vi "Alarms FGV.vi"(6 "Alarms Info":T1, 7 "Function":enum16{"Read", "Write", "Clear"}(ring)) -> (2 "Alarms Info Out":T1)   [LabVIEW 2020]
uses:
  Alarms Info Cluster.ctl
panel:
  out "error out":errorcluster
  in  "error in":errorcluster
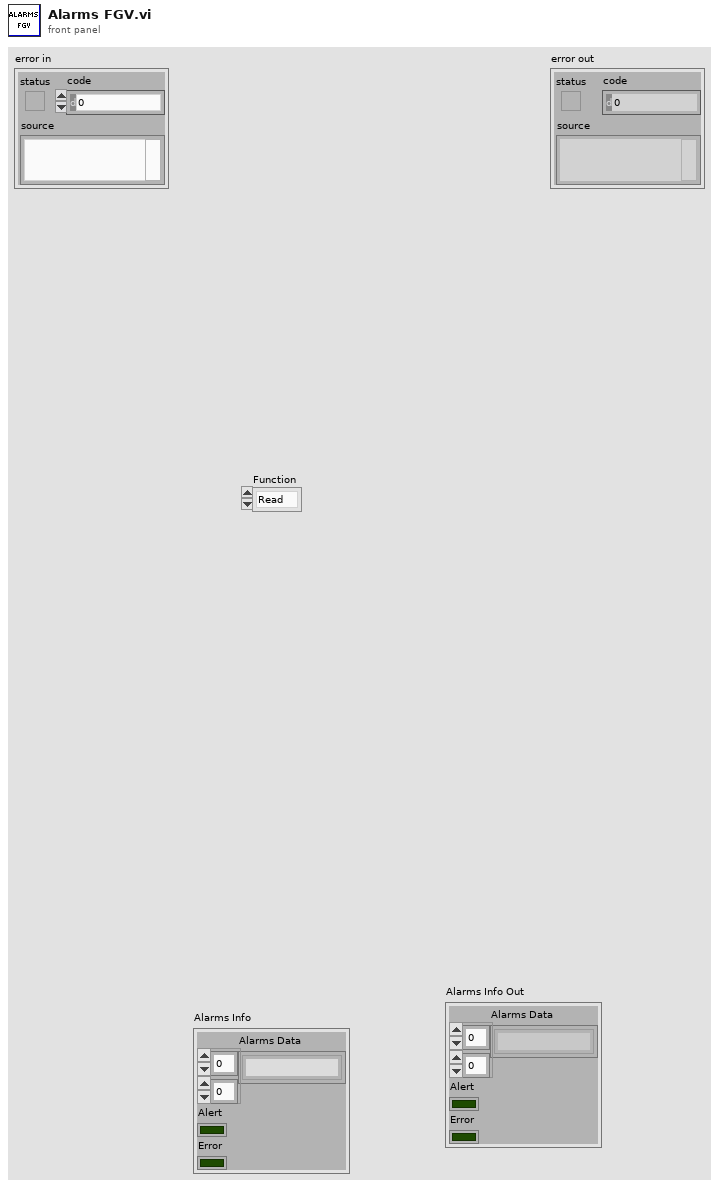
[diagram p1: front panel]
types:
  T1 = typedef "Alarms Info Cluster.ctl" = cluster{"Alarms Data":string[][], "Alert":bool, "Error":bool}
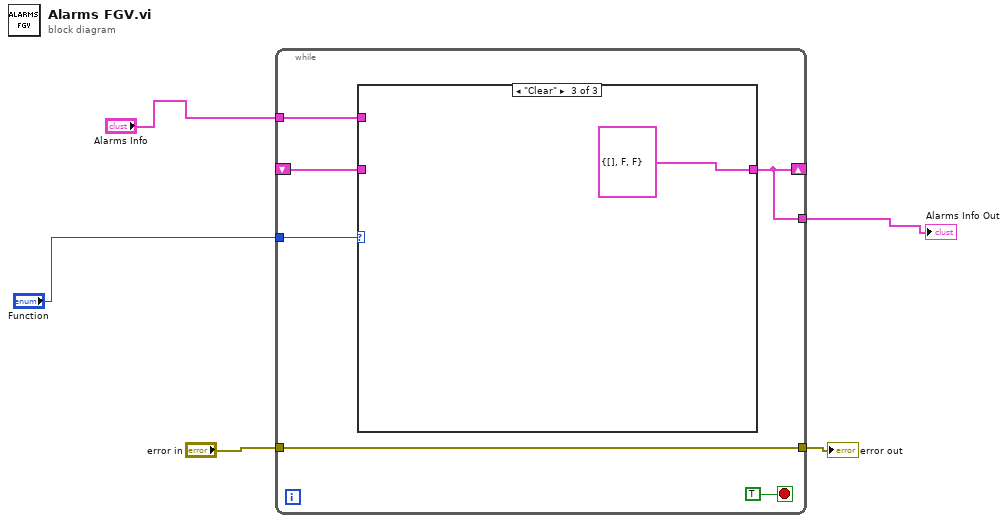
[diagram p0: block diagram]
diagram:
  n1 = while {
    tunnel: "Function" -> [w10]
    shift-right: [w7] -> _
    shift-left: _ -> [w8]
    tunnel: "Alarms Info" -> [w9]
    tunnel: [w7] -> w2
    tunnel: "error in" -> [w6]
    tunnel: [w6] -> w3
    stop <- TRUE stop-if-true
    n2 = case shown="\"Clear\"" w10 {
      tunnel: [w12 w13 T1 {"Alarms Data"=[], "Alert"=FALSE, "Error"=FALSE} ("Alarms Info Out")] -> w7
      tunnel: w9 -> [_ w13 _]
      tunnel: w8 -> [w12 _ _]
      frame "Read", Default {
      }
      frame "Write" {
      }
      frame "Clear" {
      }
    }
  }
  "error out" <- w3
  "Alarms Info Out" <- w2
